vi "Wait for keyboard.vi"(8 "error in":errorcluster, 10 "Data":variant) -> (0 "error out":errorcluster)   [LabVIEW 2025, in "Contoller.lvlib"]
doc: "This VI enqueues the named action."
uses:
  Contoller.lvlib
  Private Controls/Module Data Cluster.ctl
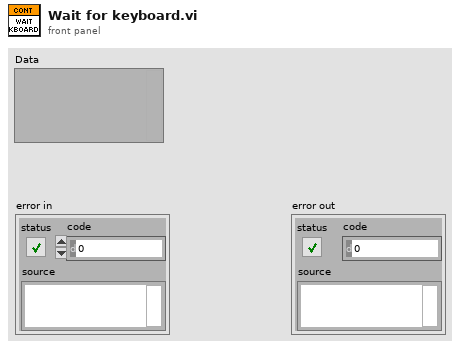
[diagram p1: front panel]
types:
  T1 = typedef "Contoller.lvlib/Module Data Cluster.ctl" = cluster{"Data":variant, "Action":enum16{"Log In Init", "Fast Cash", "New transaction", "Withdrawal Init", "Recieve Keypad", "Deposit Finish", "Balance", "Withdrawal Approved", "Terminate", "Deposit Init", "Error", "Exit", "Init", "Log In Finish", "Cancel Transaction", "Withdrawal Failed", "Cash Removed"}}
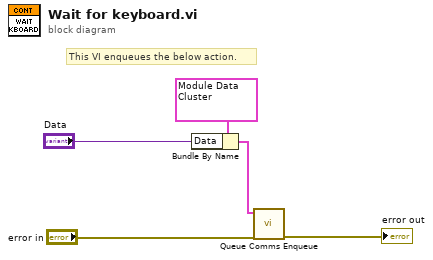
[diagram p0: block diagram]
diagram:
  # "This VI enqueues the below action."
  n1 = Bundle By Name(cluster=T1 {"Data"=variant, "Action"=enum."Fast Cash"} ("element"), "Data"="Data") -> (w2:T1)
  n2 = call "Queue Comms Enqueue.vi"("error in"="error in", "element"=w2) -> ("error out"=→"error out":errorcluster)  [unwired: 9 in]
